vi "polarimetric acquisitions.vi"(8 "error in (no error)":errorcluster, 11 "S4GEI in":refnum<class "S4GEI.lvclass">) -> (0 "error out":errorcluster, 3 "S4GEI out":refnum<class "S4GEI.lvclass">)   [LabVIEW 2018, in "S4GEI.lvclass"]
uses:
  S4GEI.lvclass
  S4GEI.lvclass/S4GEI.ctl
  State Machine/State Machine.lvclass
  Channel GUI/Channel.lvclass
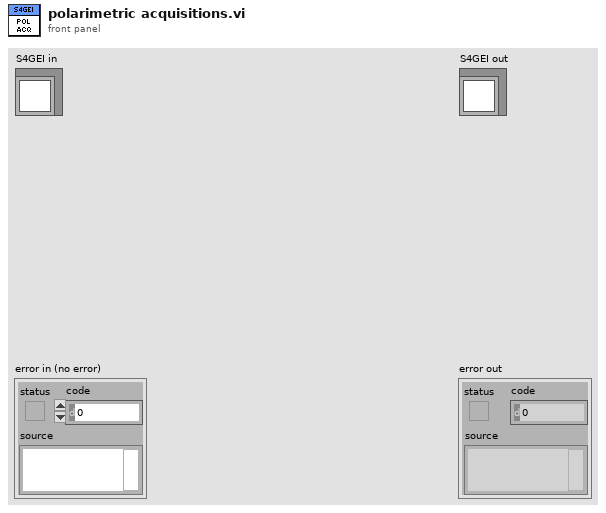
[diagram p1: front panel]
types:
  T1 = cluster{"acq finished":bool, "acq started":bool, "frames done":bool, "seqs done":bool, "cycles done":bool, "waiting exp":bool}
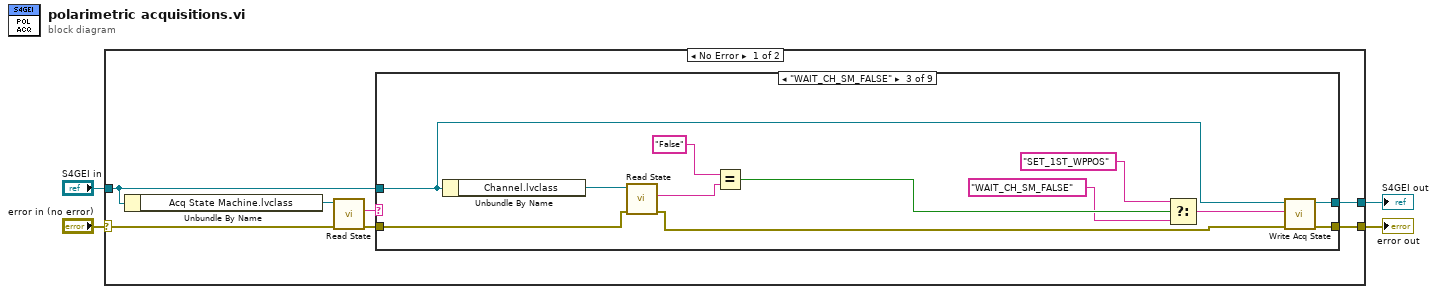
[diagram p0: block diagram]
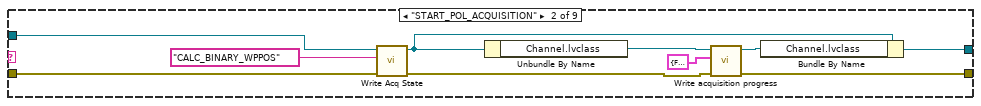
[diagram p3: hidden frame]
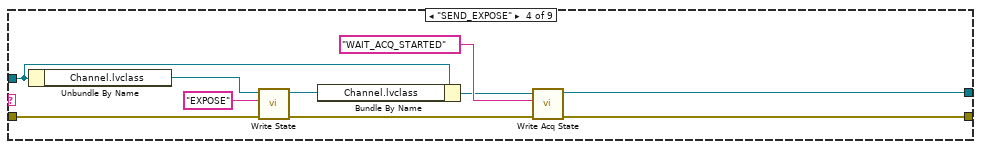
[diagram p4: hidden frame]
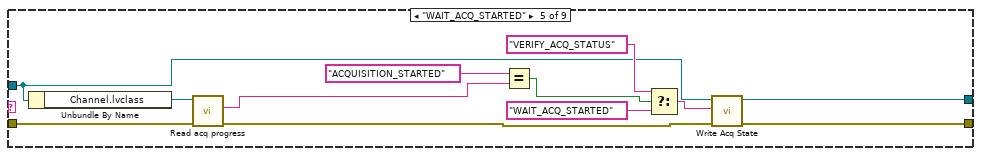
[diagram p5: hidden frame]
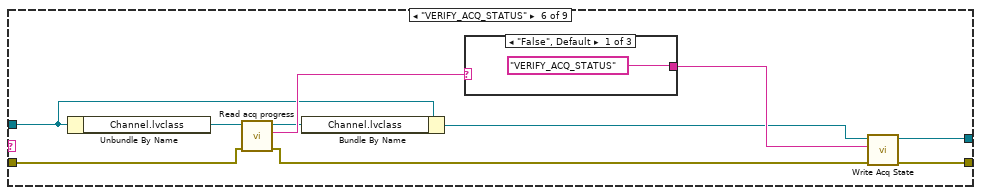
[diagram p6: hidden frame]
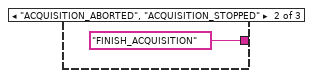
[diagram p7: hidden frame]
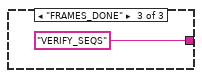
[diagram p8: hidden frame]
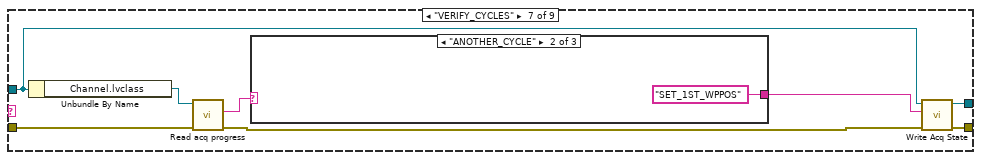
[diagram p9: hidden frame]
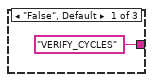
[diagram p10: hidden frame]
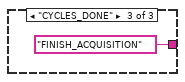
[diagram p11: hidden frame]
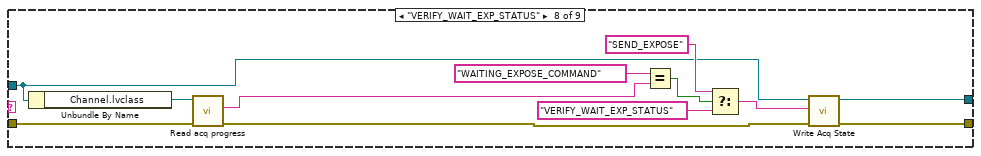
[diagram p12: hidden frame]
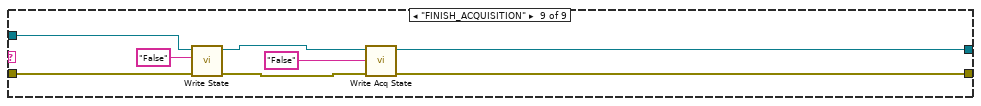
[diagram p13: hidden frame]
diagram:
  n1 = case shown="No Error" "error in (no error)" {
    selector: "error in (no error)" -> [w8 w103]
    tunnel: [w7 w103] -> w3
    tunnel: [w5 w102] -> w1
    tunnel: "S4GEI in" -> [w6 w102]
    frame No Error {
      n2 = Unbundle By Name(w6) -> ("Acq State Machine.lvclass"=w11:refnum<class "State Machine.lvclass">)
      n3 = call-dynamic "Read State.vi"("error in (no error)"=w8, "State Machine in"=w11) -> ("error out"=w9:errorcluster, "State"=w10:string)  [unwired: 7 in, 1 out]
      n4 = case shown="\"WAIT_CH_SM_FALSE\"" w10 {
        tunnel: w9 -> [w12 w21 w25 w41 w50 w61 w73 w84 w96]
        tunnel: w6 -> [w13 w22 w24 w39 w46 w60 w71 w82 w97]
        tunnel: [w13 w19 w27 w44 w48 w59 w75 w86 w95] -> w5
        tunnel: [w12 w16 w26 w43 w47 w58 w74 w85 w94] -> w7
        frame "False", Default {
        }
        frame "START_POL_ACQUISITION" {
          n5 = call "Write Acq State.vi"("error in (no error)"=w21, "State"="CALC_BINARY_WPPOS", "SPARC4_GEI in"=w22) -> ("error out"=w15:errorcluster, "SPARC4_GEI out"=w20:refnum<class "S4GEI.lvclass">)  [unwired: 7 in]
          n6 = Unbundle By Name(w20) -> ("Channel.lvclass"=w18:refnum<class "Channel.lvclass">)
          n7 = call-dynamic "Write acquisition progress.vi"("error in (no error)"=w15, "acquisition progress"=T1 {"acq finished"=FALSE, "acq started"=FALSE, "frames done"=FALSE, "seqs done"=FALSE, "cycles done"=FALSE, "waiting exp"=FALSE}, "Channel in"=w18) -> ("error out"=w16:errorcluster, "Channel out"=w17:refnum<class "Channel.lvclass">)  [unwired: 7 in]
          n8 = Bundle By Name(cluster=w20, "Channel.lvclass"=w17) -> (w19:refnum<class "S4GEI.lvclass">)
        }
        frame "WAIT_CH_SM_FALSE" {
          n9 = Unbundle By Name(w24) -> ("Channel.lvclass"=w31:refnum<class "Channel.lvclass">)
          n10 = call "Read State.vi"("error in (no error)"=w25, "Channel GEI in"=w31) -> ("error out"=w35:errorcluster, "State"=w33:string)  [unwired: 7 in, 1 out]
          n11 = Equal?(x="False" ("State"), y=w33) -> (x = y?=w34:bool)
          n12 = Select(t="SET_1ST_WPPOS" ("State"), s=w34, f="WAIT_CH_SM_FALSE" ("State")) -> (s? t:f=w32:string)
          n13 = call "Write Acq State.vi"("error in (no error)"=w35, "State"=w32, "SPARC4_GEI in"=w24) -> ("error out"=w26:errorcluster, "SPARC4_GEI out"=w27:refnum<class "S4GEI.lvclass">)  [unwired: 7 in]
        }
        frame "SEND_EXPOSE" {
          n14 = Unbundle By Name(w39) -> ("Channel.lvclass"=w42:refnum<class "Channel.lvclass">)
          n15 = call "Write State.vi"("error in (no error)"=w41, "State"="EXPOSE", "Channel GEI in"=w42) -> ("error out"=w40:errorcluster, "Channel GEI out"=w38:refnum<class "Channel.lvclass">)  [unwired: 7 in]
          n16 = Bundle By Name(cluster=w39, "Channel.lvclass"=w38) -> (w37:refnum<class "S4GEI.lvclass">)
          n17 = call "Write Acq State.vi"("error in (no error)"=w40, "State"="WAIT_ACQ_STARTED" ("f"), "SPARC4_GEI in"=w37) -> ("error out"=w43:errorcluster, "SPARC4_GEI out"=w44:refnum<class "S4GEI.lvclass">)  [unwired: 7 in]
        }
        frame "WAIT_ACQ_STARTED" {
          n18 = Unbundle By Name(w46) -> ("Channel.lvclass"=w49:refnum<class "Channel.lvclass">)
          n19 = call-dynamic "Read acq progress.vi"("error in (no error)"=w50, "Channel in"=w49) -> ("error out"=w54:errorcluster, "acq progress"=w55:string)  [unwired: 7 in, 1 out]
          n20 = Equal?(x="ACQUISITION_STARTED" ("State"), y=w55) -> (x = y?=w57:bool)
          n21 = Select(t="VERIFY_ACQ_STATUS" ("State"), s=w57, f="WAIT_ACQ_STARTED" ("State")) -> (s? t:f=w51:string)
          n22 = call "Write Acq State.vi"("error in (no error)"=w54, "State"=w51, "SPARC4_GEI in"=w46) -> ("error out"=w47:errorcluster, "SPARC4_GEI out"=w48:refnum<class "S4GEI.lvclass">)  [unwired: 7 in]
        }
        frame "VERIFY_ACQ_STATUS" {
          n23 = Unbundle By Name(w60) -> ("Channel.lvclass"=w63:refnum<class "Channel.lvclass">)
          n24 = call-dynamic "Read acq progress.vi"("error in (no error)"=w61, "Channel in"=w63) -> ("error out"=w65:errorcluster, "acq progress"=w66:string, "Channel out"=w64:refnum<class "Channel.lvclass">)  [unwired: 7 in]
          n25 = Bundle By Name(cluster=w60, "Channel.lvclass"=w64) -> (w62:refnum<class "S4GEI.lvclass">)
          n26 = case shown="\"False\", Default" w66 {
            tunnel: ["VERIFY_ACQ_STATUS" "FINISH_ACQUISITION" "VERIFY_SEQS"] -> w67
            frame "False", Default {
            }
            frame "ACQUISITION_ABORTED", "ACQUISITION_STOPPED" {
            }
            frame "FRAMES_DONE" {
            }
          }
          n27 = call "Write Acq State.vi"("error in (no error)"=w65, "State"=w67, "SPARC4_GEI in"=w62) -> ("error out"=w58:errorcluster, "SPARC4_GEI out"=w59:refnum<class "S4GEI.lvclass">)  [unwired: 7 in]
        }
        frame "VERIFY_CYCLES" {
          n28 = Unbundle By Name(w71) -> ("Channel.lvclass"=w72:refnum<class "Channel.lvclass">)
          n29 = call-dynamic "Read acq progress.vi"("error in (no error)"=w73, "Channel in"=w72) -> ("error out"=w76:errorcluster, "acq progress"=w77:string)  [unwired: 7 in, 1 out]
          n30 = case shown="\"ANOTHER_CYCLE\"" w77 {
            tunnel: ["VERIFY_CYCLES" ("State") "SET_1ST_WPPOS" ("y") "FINISH_ACQUISITION" ("State")] -> w78
            frame "False", Default {
            }
            frame "ANOTHER_CYCLE" {
            }
            frame "CYCLES_DONE" {
            }
          }
          n31 = call "Write Acq State.vi"("error in (no error)"=w76, "State"=w78, "SPARC4_GEI in"=w71) -> ("error out"=w74:errorcluster, "SPARC4_GEI out"=w75:refnum<class "S4GEI.lvclass">)  [unwired: 7 in]
        }
        frame "VERIFY_WAIT_EXP_STATUS" {
          n32 = Unbundle By Name(w82) -> ("Channel.lvclass"=w83:refnum<class "Channel.lvclass">)
          n33 = call-dynamic "Read acq progress.vi"("error in (no error)"=w84, "Channel in"=w83) -> ("error out"=w91:errorcluster, "acq progress"=w93:string)  [unwired: 7 in, 1 out]
          n34 = Equal?(x="WAITING_EXPOSE_COMMAND", y=w93) -> (x = y?=w90:bool)
          n35 = Select(t="SEND_EXPOSE" ("x"), s=w90, f="VERIFY_WAIT_EXP_STATUS" ("x")) -> (s? t:f=w89:string)
          n36 = call "Write Acq State.vi"("error in (no error)"=w91, "State"=w89, "SPARC4_GEI in"=w82) -> ("error out"=w85:errorcluster, "SPARC4_GEI out"=w86:refnum<class "S4GEI.lvclass">)  [unwired: 7 in]
        }
        frame "FINISH_ACQUISITION" {
          n37 = call "Write State.vi"("error in (no error)"=w96, "State"="False", "SPARC4_GEI in"=w97) -> ("error out"=w99:errorcluster, "SPARC4_GEI out"=w98:refnum<class "S4GEI.lvclass">)  [unwired: 7 in]
          n38 = call "Write Acq State.vi"("error in (no error)"=w99, "State"="False", "SPARC4_GEI in"=w98) -> ("error out"=w94:errorcluster, "SPARC4_GEI out"=w95:refnum<class "S4GEI.lvclass">)  [unwired: 7 in]
        }
      }
    }
    frame Error {
    }
  }
  "error out" <- w3
  "S4GEI out" <- w1
